vi "Write XY graph ref.vi"(8 "error in (no error)":errorcluster, 10 "XY graph ref":refnum<vi>, 11 "Cursor Digitizer in":refnum<class "Cursor Digitizer.lvclass">) -> (0 "error out":errorcluster, 3 "Cursor Digitizer out":refnum<class "Cursor Digitizer.lvclass">)   [LabVIEW 2019, in "Cursor Digitizer.lvclass"]
uses:
  Cursor Digitizer.lvclass
  Cursor Digitizer.lvclass/Cursor Digitizer.ctl
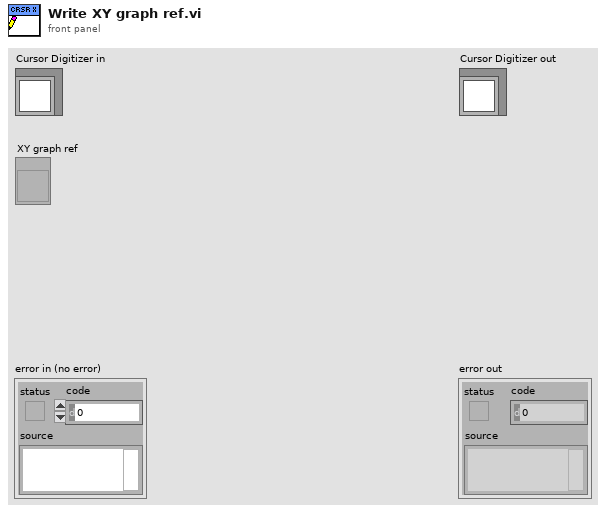
[diagram p1: front panel]
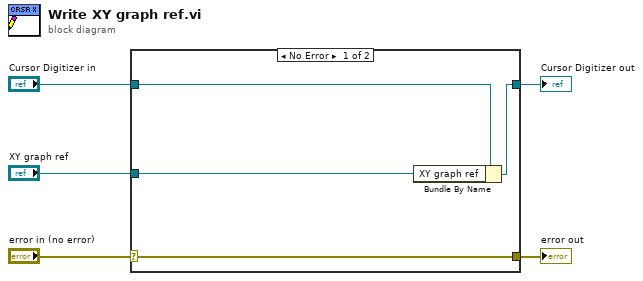
[diagram p0: block diagram]
diagram:
  n1 = case shown="No Error" "error in (no error)" {
    selector: "error in (no error)" -> [w9 w10]
    tunnel: [w9 w10] -> w4
    tunnel: [w7 w11] -> w2
    tunnel: "Cursor Digitizer in" -> [w8 w11]
    tunnel: "XY graph ref" -> [w6 _]
    frame No Error {
      n2 = Bundle By Name(cluster=w8, "XY graph ref"=w6) -> (w7:refnum<class "Cursor Digitizer.lvclass">)
    }
    frame Error {
    }
  }
  "error out" <- w4
  "Cursor Digitizer out" <- w2
